vi "FMA1600A Send Receive.vi"(7 "Unit ID":string, 8 "error in (no error)":errorcluster, 9 "Gas Type":T1, 10 "FMA1600A Commands":T2, 11 "VISA Refnum in":refnum<visa-resource-name>) -> (0 "error out":errorcluster, 2 "Raw FMA1600A Data":string, 3 "VISA Refnum out":refnum<visa-resource-name>)   [LabVIEW 2016]
uses:
  Type Definitions/FMA1600A Commands.ctl
  Type Definitions/FMA1600A Gas Type.ctl
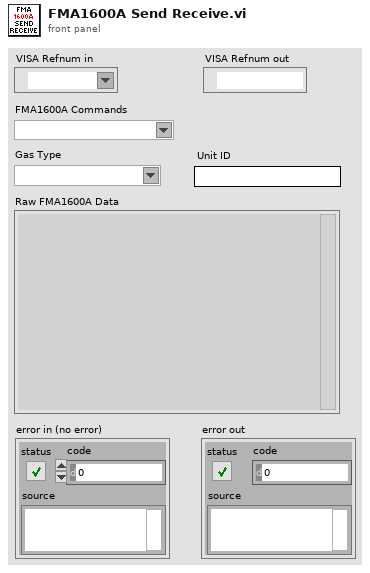
[diagram p1: front panel]
types:
  T1 = typedef "FMA1600A Gas Type.ctl" = string
  T2 = typedef "FMA1600A Commands.ctl" = string
  T3 = typedef "FMA1600A Data.ctl" = cluster{"Pressure (PSIA)":dbl, "Temperature (°F)":dbl, "Vol. Flow (LPM)":dbl, "Mass Flow (SLPM)":dbl, "Gas Type":string, "Tot. Flow (Liters)":dbl, "Meter ID":string}
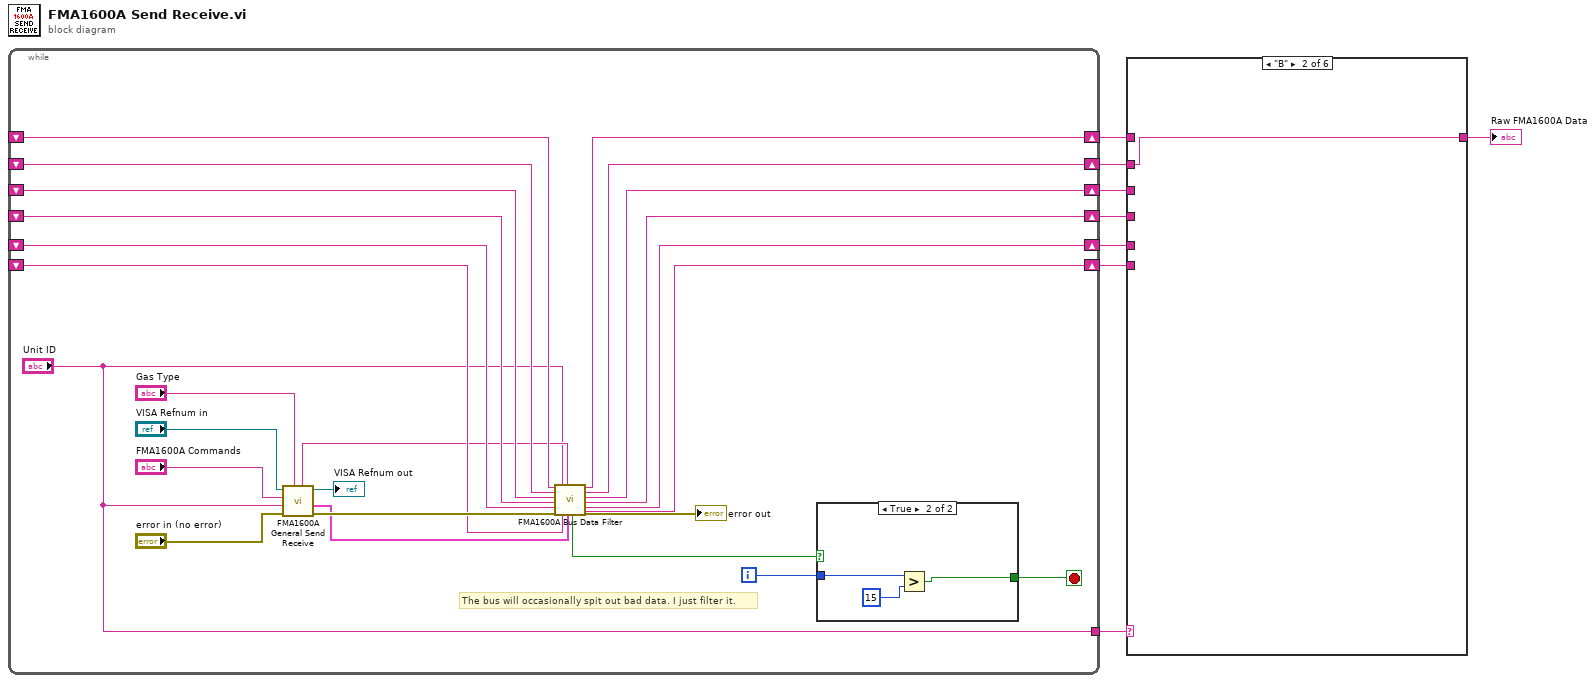
[diagram p0: block diagram]
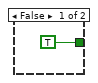
[diagram p7: hidden frame]
diagram:
  n1 = while {
    shift-right: [w23] -> w7
    shift-left: _ -> [w24]
    shift-right: [w21] -> w5
    shift-left: _ -> [w22]
    shift-right: [w20] -> w4
    shift-left: _ -> [w19]
    shift-right: [w17] -> w3
    shift-left: _ -> [w18]
    shift-right: [w15] -> w2
    shift-left: _ -> [w16]
    shift-right: [w13] -> w1
    shift-left: _ -> [w14]
    tunnel: ["Unit ID"] -> w8
    i -> [w29]
    stop <- w28 stop-if-true
    # "The bus will occasionally spit out bad data. I just filter it."
    n2 = call "FMA1600A General Send Receive.vi"("Gas Type"="Gas Type", "error in (no error)"="error in (no error)", "Unit ID in"="Unit ID", "FMA1600A Commands"="FMA1600A Commands", "VISA Refnum in"="VISA Refnum in") -> ("error out"=w26:errorcluster, "FMA1600A Gas Data"=w12:T3, "VISA Refnum out"=→"VISA Refnum out":refnum<visa-resource-name>, "Data Stream"=w11:string)  [unwired: 3 in]
    n3 = call "FMA1600A Bus Data Filter.vi"("Station A Input"=w24, "Station B Input"=w22, "Station C Input"=w19, "Station D Input"=w18, "Station E Input"=w16, "Error In"=w26, "Unit ID"="Unit ID", "Station F Input"=w14, "Data Stream"=w11, "FMA1600A Gas Data"=w12) -> ("Check Shutdown"=w10:bool, "Station F Output"=w13:string, "Station A Output"=w23:string, "Station B Output"=w21:string, "Station C Output"=w20:string, "Station D Output"=w17:string, "Station E Output"=w15:string, "Error Out"=→"error out":errorcluster)  [unwired: 2 in]
    n4 = case shown="True" w10 {
      tunnel: [TRUE ("y") w35] -> w28
      tunnel: w29 -> [_ w36]
      frame False {
      }
      frame True {
        n5 = Greater?(x=w36, y=15) -> (0:w35:bool)
      }
    }
  }
  n6 = case shown="\"B\"" w8 {
    tunnel: [w38 w39 w40 w41 w42 w43] -> w6
    tunnel: w7 -> [w38 _ _ _ _ _]
    tunnel: w5 -> [_ w39 _ _ _ _]
    tunnel: w4 -> [_ _ w40 _ _ _]
    tunnel: w3 -> [_ _ _ w41 _ _]
    tunnel: w2 -> [_ _ _ _ w42 _]
    tunnel: w1 -> [_ _ _ _ _ w43]
    frame "A", Default {
    }
    frame "B" {
    }
    frame "C" {
    }
    frame "D" {
    }
    frame "E" {
    }
    frame "F" {
    }
  }
  "Raw FMA1600A Data" <- w6
